vi "Runner.vi"(8 "error in (no error)":errorcluster, 10 "Runnable":refnum<class "Runnable.lvclass">, 11 "Parallell Test Runner In":refnum<class "Parallell Test Runner.lvclass">) -> (0 "error out":errorcluster)   [LabVIEW 2020, in "Parallell Test Runner.lvclass"]
uses:
  Parallell Test Runner.lvclass
  Core/Runnable/Runnable.lvclass
  API/LUnit Test Suite/LUnit Test Suite.lvclass
  Parallell Test Runner.lvclass/Parallell Test Runner.ctl
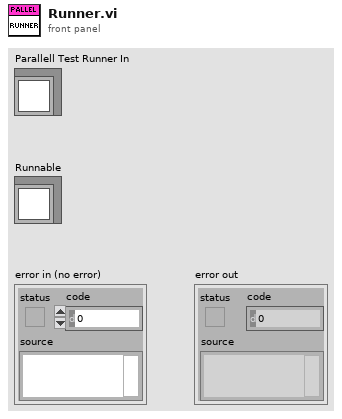
[diagram p1: front panel]
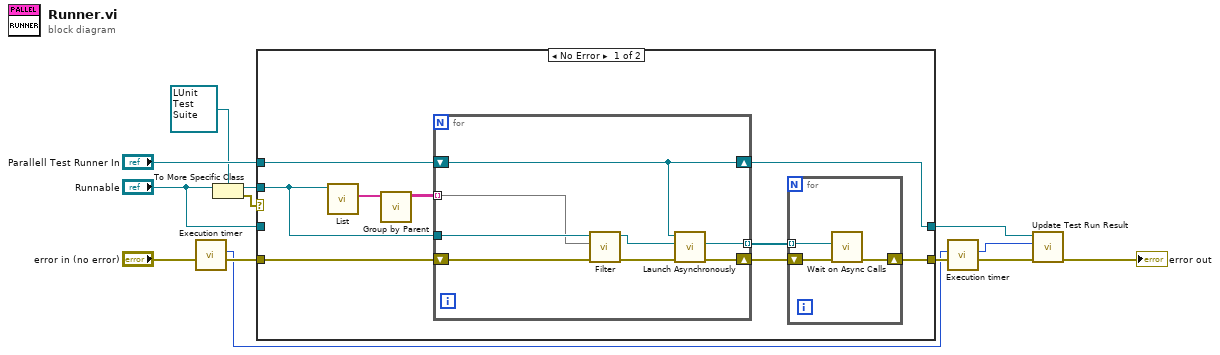
[diagram p0: block diagram]
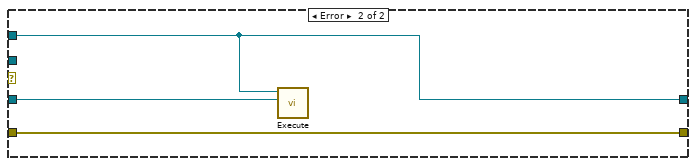
[diagram p2: hidden frame]
diagram:
  n1 = call "Execution timer.vi"("error in (no error)"="error in (no error)") -> ("error out"=w11:errorcluster, "Current or Duration [ms]"=w7:u32)  [unwired: 9 in]
  n2 = To More Specific Class(target class=refnum<class "LUnit Test Suite.lvclass"> refnum, reference="Runnable") -> (specific class reference=w5:refnum<class "LUnit Test Suite.lvclass">, error out=w3:errorcluster)  [unwired: 1 in]
  n3 = case shown="No Error" w3 {
    tunnel: "Parallell Test Runner In" -> [w18 w36]
    tunnel: w11 -> [w17 w34]
    tunnel: [w16 w34] -> w10
    tunnel: w5 -> [w15 _]
    tunnel: [w14 w36] -> w2
    tunnel: "Runnable" -> [_ w35]
    frame No Error {
      n4 = call "List.vi"("LUnit Test Suite In"=w15) -> ("List of Runnables"=w22:string[])  [unwired: 9 in, 1 out]
      n5 = call "Group by Parent.vi"("List of Runnables"=w22) -> ("Method Groups"=w21:string[][])  [unwired: 10 in]
      n6 = for {
        tunnel: w15 -> [w30]
        shift-right: [w29] -> w20
        shift-left: w17 -> [w28]
        tunnel: w21 -> [w26] mode=indexing
        tunnel: [w24] -> w19 mode=indexing
        shift-right: [w23] -> w14
        shift-left: w18 -> [w23]
        n7 = call "Filter.vi"("error in (no error)"=w28, "Selected Runnables"=w26, "LUnit Test Suite In"=w30) -> ("error out"=w27:errorcluster, "LUnit Test Suite Out"=w25:refnum<class "LUnit Test Suite.lvclass">)  [unwired: 7 in]
        n8 = call "Launch Asynchronously.vi"("error in (no error)"=w27, "Runnable in"=w25, "Parallell Test Runner In"=w23) -> ("error out"=w29:errorcluster, "reference out"=w24:refnum<vi>)  [unwired: 7 in]
      }
      n9 = for {
        shift-right: [w32] -> w16
        shift-left: w20 -> [w33]
        tunnel: w19 -> [w31] mode=indexing
        n10 = call "Wait on Async Calls.vi"("error in (no error)"=w33, "reference out"=w31) -> ("error out"=w32:errorcluster)  [unwired: 9 in]
      }
    }
    frame Error {
      n11 = call "Execute.vi"("Runnable"=w35, "Parallell Test Runner In"=w36) -> ()  [unwired: 10 in]
    }
  }
  n12 = call "Execution timer.vi"("error in (no error)"=w10, "millisecond timer value"=w7) -> ("error out"=w8:errorcluster, "Current or Duration [ms]"=w6:u32)  [unwired: 8 in]
  n13 = call "Update Test Run Result.vi"("error in (no error)"=w8, "Duration [ms]"=w6, "Single Thread Test Runner in"=w2) -> ("error out"=→"error out":errorcluster)  [unwired: 8 in]
